vi "Untitled 2.vi"() -> ()   [LabVIEW 2013]
uses:
  <vilib>/rvi/DataTransferAndStorage/Container/XNode/niFpgaContainer.xnode
  <vilib>/rvi/Memory/Memory_Emulation/nirvimemoryFastEmulation.vi
  <vilib>/rvi/Memory/Memory_Emulation/nirvimemoryEmulation.vi
panel:
  out "Waveform Graph 4":i16[](graph)
  out "Waveform Graph 3":u32[](graph)
  out "Waveform Graph 2":i16[](graph)
  out "Waveform Graph":u32[](graph)
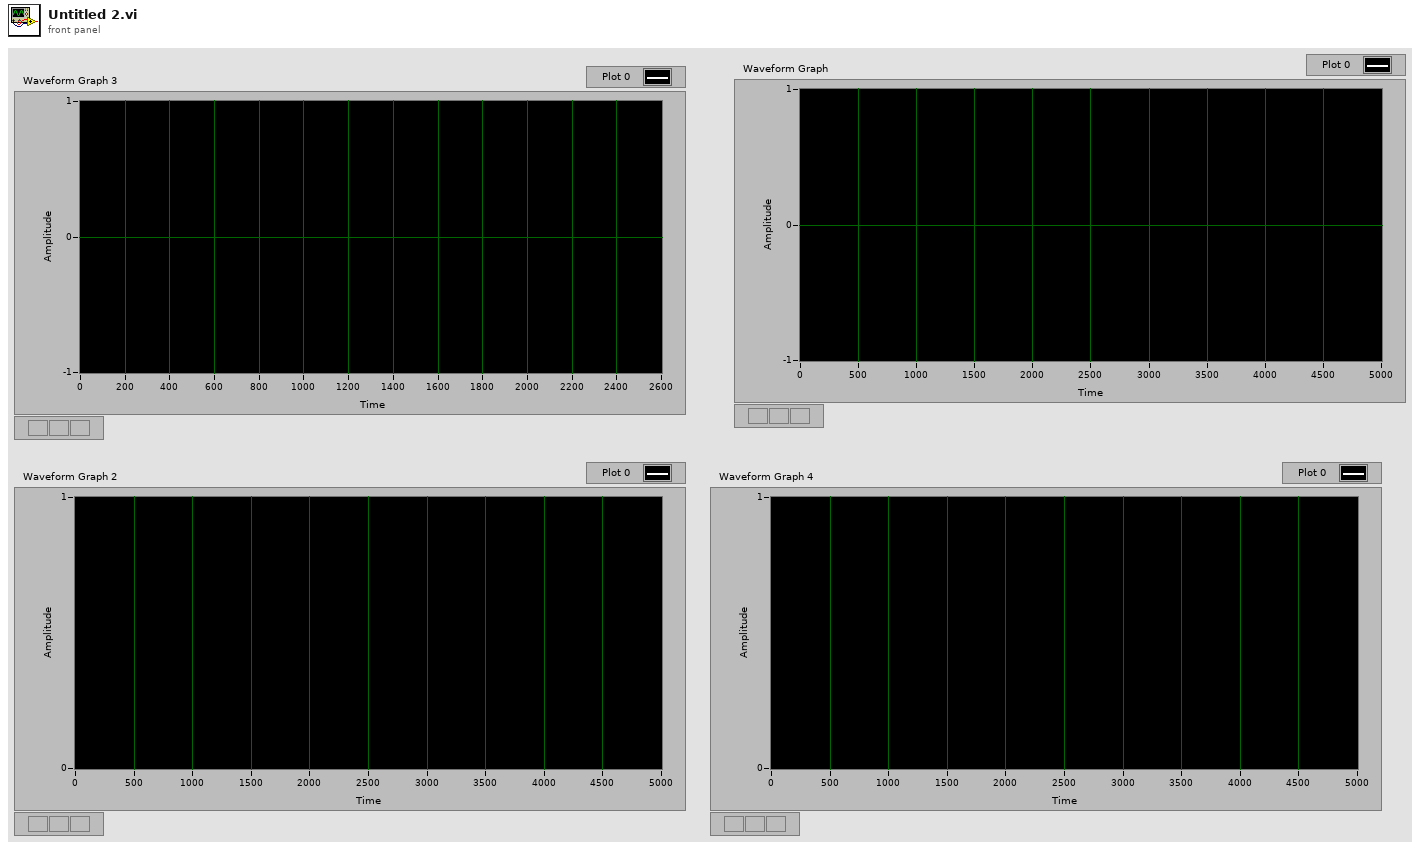
[diagram p1: front panel]
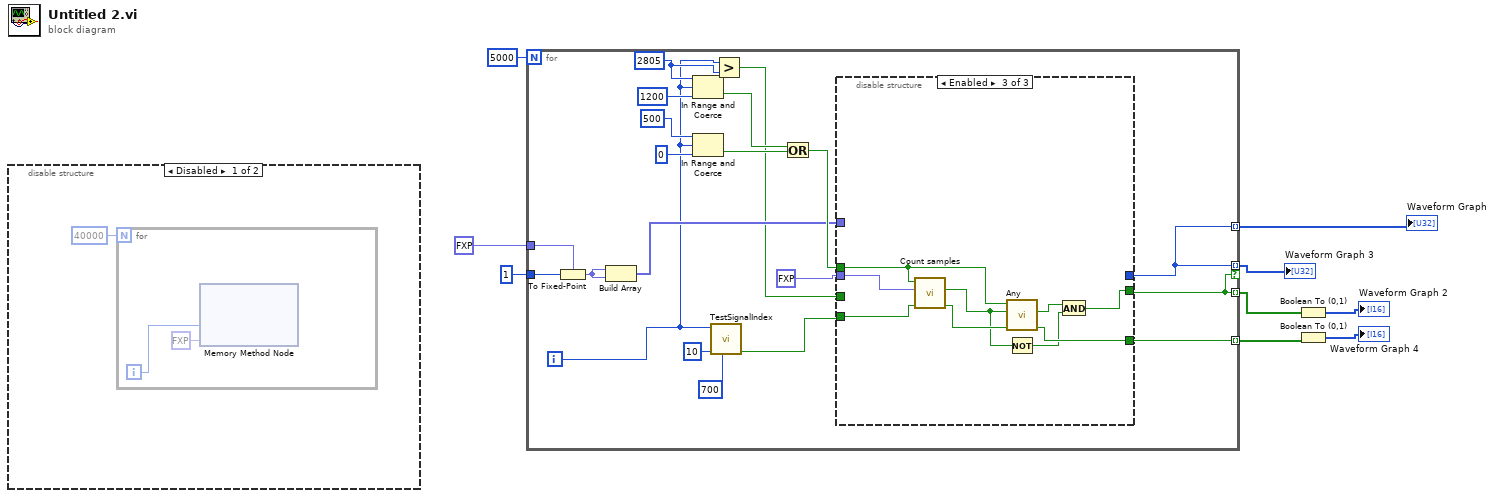
[diagram p0: block diagram]
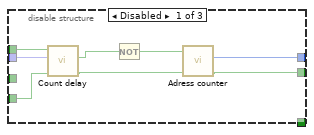
[diagram p3: hidden frame]
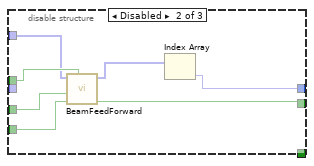
[diagram p4: hidden frame]
diagram:
  n1 = disable-structure shown="Disabled" {
    frame Disabled {
      n2 = for {
        N: 40000 -> [_]
        i -> [w12]
        n3 = xnode ("Memory Method Node")("Address"=w12, "Data"=fxp<+/-,16,14> 17.0) -> ()  [unwired: 1 in, 1 out]
      }
    }
    frame Enabled {
    }
  }
  n4 = for {
    N: 5000 -> [_]
    tunnel: [w25] -> w5 mode=indexing if=w24
    tunnel: [w24] -> w7 mode=indexing
    tunnel: [w25] -> w6 mode=indexing
    tunnel: fxp<+/-,16,14> 0.0 ("Q in") -> [w21]
    tunnel: 1 -> [w18]
    tunnel: [w13] -> w1 mode=indexing
    i -> [w15]
    w16 = 2805 ("y")
    n5 = To Fixed-Point(fixed-point type=w21, number=w18) -> (fixed-point=w20:fxp<+/-,16,14>)
    n6 = Build Array(w20, w20) -> (w19:fxp<+/-,16,14>[])
    n7 = In Range and Coerce(upper limit=w16, x=w15, lower limit=1200 ("y")) -> (In Range?=w17:bool)  [unwired: 1 out]
    n8 = In Range and Coerce(upper limit=500 ("y"), x=w15, lower limit=0 ("y")) -> (In Range?=w22:bool)  [unwired: 1 out]
    n9 = call "TestSignalIndex.vi"("initial delay"=700, "cycles per sample"=10, "index"=w15) -> ("valid out"=w23:bool)  [unwired: 7 in, 1 out]
    n10 = Greater?(x=w15, y=w16) -> (0:w14:bool)
    n11 = Or(x=w17, y=w22) -> (x .or. y?=w26:bool)
    n12 = disable-structure shown="Enabled" {
      disable-tunnel: fxp<+/-,16,16> 10.0 ("Count to skip") -> [w40 _ w56]
      disable-tunnel: w26 -> [w39 w47 w52]
      disable-tunnel: [w36 w42 _] -> w25
      disable-tunnel: [w35 w41 w48] -> w24
      disable-tunnel: w23 -> [w34 w46 w55]
      disable-tunnel: w14 -> [_ w45 _]
      disable-tunnel: w19 -> [_ w44 _]
      disable-tunnel: [_ _ w53] -> w13
      frame Disabled {
        n13 = call "Count delay.vi"("input valid"=w34, "Count to skip"=w40, "Reset"=w39) -> ("output valid"=w33:bool, "count done?"=w38:bool)  [unwired: 7 in]
        n14 = Not(x=w38) -> (.not. x?=w37:bool)
        n15 = call "Adress counter.vi"("input valid"=w33, "Reset"=w37) -> ("output valid"=w35:bool, "Address"=w36:u32)  [unwired: 8 in]
      }
      frame Disabled {
        n16 = call "BeamFeedForward.vi"("Reset"=w47, "input valid"=w46, "beam enabled"=w45, "Data in"=w44) -> ("output valid"=w41:bool, "Data out"=w43:fxp<+/-,16,14>[])  [unwired: 4 in, 2 out]
        n17 = Index Array(array=w43) -> (element=w42:fxp<+/-,16,14>)  [unwired: 1 in]
      }
      frame Enabled {
        n18 = call "Count samples.vi"("input valid"=w55, "Samples to count"=w56, "Reset"=w52) -> ("output valid"=w54:bool, "counting"=w51:bool)  [unwired: 7 in]
        n19 = call "Any.vi"("input valid"=w54, "Value"=w51, "Reset"=w52) -> ("output valid"=w53:bool, "Any?"=w50:bool)  [unwired: 7 in]
        n20 = Not(x=w51) -> (.not. x?=w49:bool)
        n21 = And(x=w50, y=w49) -> (x .and. y?=w48:bool)
      }
    }
  }
  "Waveform Graph" <- w6
  "Waveform Graph 3" <- w5
  n22 = Boolean To (0,1)(Boolean=w7) -> (0, 1=→"Waveform Graph 2":i16[])
  n23 = Boolean To (0,1)(Boolean=w1) -> (0, 1=→"Waveform Graph 4":i16[])
